vi "Create Label Name.vi"(10 "label number":u8, 11 "label XML name":string) -> (3 "label name":string)   [LabVIEW 2016]
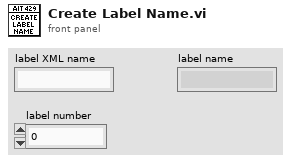
[diagram p1: front panel]
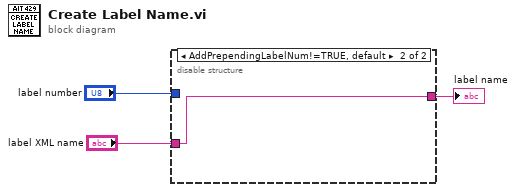
[diagram p0: block diagram]
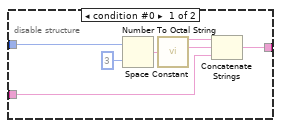
[diagram p2: hidden frame]
diagram:
  n1 = disable-structure shown="AddPrependingLabelNum!=TRUE, default" {
    disable-tunnel: "label XML name" -> [w9 w10]
    disable-tunnel: [w8 w10] -> w2
    disable-tunnel: "label number" -> [w7 _]
    frame condition #0 {
      n2 = Number To Octal String(1:i16 3 ("width (-)"), 2:w7) -> (0:w5:string)
      n3 = call <vilib>:"Space Constant.vi"() -> ("String"=w6:string)
      n4 = Concatenate Strings(w5, w6, w9) -> (w8:string)
    }
    frame condition #1 (active) {
    }
  }
  "label name" <- w2
